vi "VoltageUpdate.Write Configuration File.vi"(8 "error in (no error)":errorcluster, 10 "Configuration":T1, 11 "VoltageUpdate":refnum<class "VoltageUpdate.lvclass">) -> (0 "error out":errorcluster, 3 "VoltageUpdate out":refnum<class "VoltageUpdate.lvclass">)   [LabVIEW 2016, in "VoltageUpdate.lvclass"]
uses:
  VoltageUpdate.lvclass
  C:/Program Files (x86)/National Instruments/LabVIEW 2016/user.lib/LevyLab/Levylab Instruments/SMOs/Instrument/Instrument.lvclass
  Typedefs/VoltageUpdate.Configuration--Cluster.ctl
  <userlib>/LevyLab/Levylab Instruments/SMOs/Instrument/Instrument.lvclass/Instrument.ctl
  <userlib>/LevyLab/Levylab Instruments/SMOs/Configuration/Configuration.lvclass
  <userlib>/LevyLab/Levylab Instruments/SMOs/Instrument/Instrument.lvclass
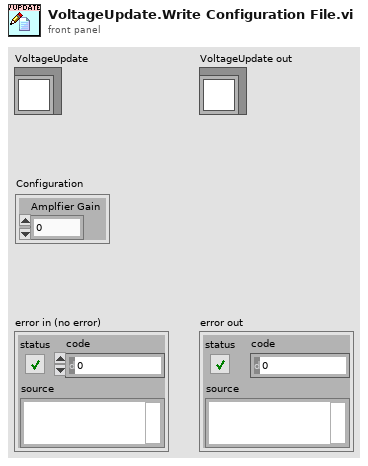
[diagram p1: front panel]
types:
  T1 = typedef "VoltageUpdate.lvclass/VoltageUpdate.Configuration--Cluster.ctl" = cluster{"Amplfier Gain":dbl}
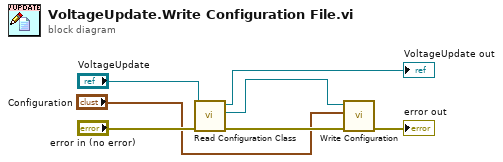
[diagram p0: block diagram]
diagram:
  n1 = call <userlib>:"Read Configuration Class.vi"("error in (no error)"="error in (no error)", "Instrument in"="VoltageUpdate") -> ("error out"=w3:errorcluster, "Configuration.lvclass"=w6:refnum<class "Configuration.lvclass">, "Instrument out"=→"VoltageUpdate out":refnum<class "VoltageUpdate.lvclass">)  [unwired: 7 in]
  n2 = call <userlib>:"Write Configuration.vi"("error in (no error)"=w3, "Variant"="Configuration", "Configuration in"=w6) -> ("error out"=→"error out":errorcluster)  [unwired: 7 in, 1 out]
